vi "CThread Get Loop Count.vi"   [LabVIEW 2012, in "CThread.lvlib"]
uses:
  CThread.lvlib
  XNodes/terminalnode/CThread VI Terminal Node.xnode
  Base/CThread Base - Get Loop Count.vi
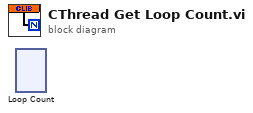
[diagram p0: block diagram]
diagram:
  n1 = xnode "Loop Count"() -> ()  [unwired: 1 in, 2 out]
